vi "CRYCheck Statistic Data.vi"(8 "Results":string[](array[string]), 9 "Curves":string[](array[string]), 11 "No.VI":i32) -> (0 "Result Out":T1[](array[typedef]) {"Margin" format="%.2f"}, 2 "Data Out":T2 {"Z data" items=["dB", "Lin"]; "X data" items=["dB", "Lin"]; "Y data" items=["dB", "Lin"]; "Z dB ref" format="%.1f"; "Z axis" items=["Log", "Lin"]; "X dB ref" format="%.1f"; "X axis" items=["Log", "Lin"]; "Y axis" items=["Log", "Lin"]; "Y dB ref" format="%.1f"; "Curve"."z" format="%.2f"; "Curve"."y" format="%.2f"; "Curve"."x" format="%.2f"})   [LabVIEW 2013]
uses:
  Typedef Control/CRYData Cluster Array.ctl
  Typedef Control/CRYData Cluster.ctl
  Typedef Control/CRYResult Cluster.ctl
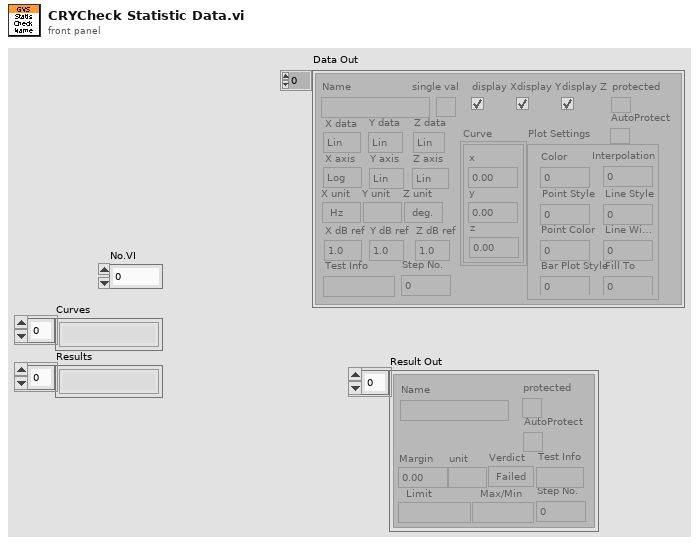
[diagram p1: front panel]
types:
  T1 = typedef "CRYResult Cluster.ctl" = cluster{"Name":string, "Margin":dbl, "unit":string, "Verdict":bool, "Limit":string, "Max/Min":string, "protected":bool, "Step No.":i32, "Test Info":string, "AutoProtect":bool}
  T2 = typedef "CRYData Cluster Array.ctl" = T3[]
  T3 = typedef "CRYData Cluster.ctl" = cluster{"Name":string, "Curve":cluster{"x":dbl, "y":dbl, "z":dbl}[], "X data":u16, "Y data":u16, "Z data":u16, "X axis":u16, "Y axis":u16, "Z axis":u16, "X unit":string, "Y unit":string, "Z unit":string, "X dB ref":dbl, "Y dB ref":dbl, "Z dB ref":dbl, "single val":bool, "protected":bool, "display X":bool, "display Y":bool, "display Z":bool, "Test Info":string, "Step No.":i32, "Plot Settings":cluster{"Color":u32, "Interpolation":u8, "Point Style":u8, "Line Style":u8, "Point Color":u32, "Line Width":u8, "Bar Plot Style":u8, "Fill To":i16}, "AutoProtect":bool}
  T4 = typedef "CRYResult Cluster Array.ctl" = T1[]
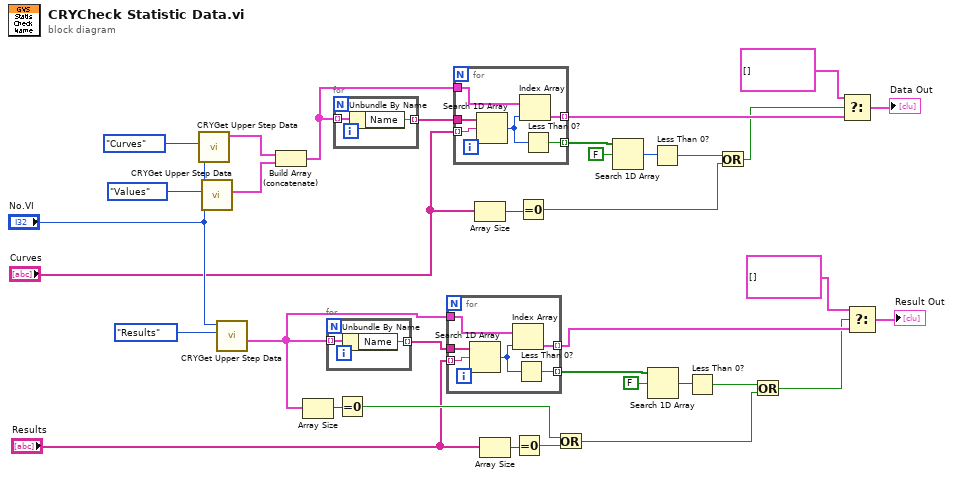
[diagram p0: block diagram]
diagram:
  n1 = call "CRYGet Upper Step Data.vi"("Type In"=enum16{"Curves", "Values", "Results", "WFM"}."Curves", "No.VI"="No.VI") -> ("Curve array"=w29:T2)  [unwired: 9 out]
  n2 = call "CRYGet Upper Step Data.vi"("Type In"=enum16{"Curves", "Values", "Results", "WFM"}."Values", "No.VI"="No.VI") -> ("Value array"=w28:T2)  [unwired: 9 out]
  n3 = call "CRYGet Upper Step Data.vi"("Type In"=enum16{"Curves", "Values", "Results", "WFM"}."Results", "No.VI"="No.VI") -> ("Result array"=w11:T4)  [unwired: 9 out]
  n4 = Build Array (concatenate)(w29, w28) -> (w26:T2)
  n5 = Array Size(array=w11) -> (size(s)=w12:i32)
  n6 = for {
    tunnel: w11 -> [w37] mode=indexing
    tunnel: [w36] -> w10 mode=indexing
    n7 = Unbundle By Name(w37) -> ("Name"=w36:string)
  }
  n8 = for {
    tunnel: w26 -> [w39] mode=indexing
    tunnel: [w38] -> w27 mode=indexing
    n9 = Unbundle By Name(w39) -> ("Name"=w38:string)
  }
  n10 = Equal To 0?(x=w12) -> (x = 0?=w13:bool)
  n11 = for {
    tunnel: "Results" -> [w45] mode=indexing
    tunnel: w10 -> [w44]
    tunnel: w11 -> [w43]
    tunnel: [w42] -> w4 mode=indexing
    tunnel: [w40] -> w5 mode=indexing
    n12 = Search 1D Array(1D array=w44, element=w45) -> (index of element=w41:i32)  [unwired: 1 in]
    n13 = Index Array(array=w43, index=w41) -> (element=w42:T1)
    n14 = Less Than 0?(x=w41) -> (x < 0?=w40:bool)
  }
  n15 = for {
    tunnel: "Curves" -> [w51] mode=indexing
    tunnel: w27 -> [w50]
    tunnel: w26 -> [w49]
    tunnel: [w48] -> w34 mode=indexing
    tunnel: [w46] -> w22 mode=indexing
    n16 = Search 1D Array(1D array=w50, element=w51) -> (index of element=w47:i32)  [unwired: 1 in]
    n17 = Index Array(array=w49, index=w47) -> (element=w48:T3)
    n18 = Less Than 0?(x=w47) -> (x < 0?=w46:bool)
  }
  n19 = Array Size(array="Curves") -> (size(s)=w16:i32)
  n20 = Array Size(array="Results") -> (size(s)=w15:i32)
  n21 = Equal To 0?(x=w15) -> (x = 0?=w14:bool)
  n22 = Equal To 0?(x=w16) -> (x = 0?=w7:bool)
  n23 = Or(x=w13, y=w14) -> (x .or. y?=w6:bool)
  n24 = Search 1D Array(1D array=w22, element=FALSE) -> (index of element=w24:i32)  [unwired: 1 in]
  n25 = Search 1D Array(1D array=w5, element=FALSE) -> (index of element=w20:i32)  [unwired: 1 in]
  n26 = Less Than 0?(x=w24) -> (x < 0?=w23:bool)
  n27 = Less Than 0?(x=w20) -> (x < 0?=w21:bool)
  n28 = Or(x=w23, y=w7) -> (x .or. y?=w18:bool)
  n29 = Or(x=w21, y=w6) -> (x .or. y?=w3:bool)
  n30 = Select(t=T2 [] ("Data in"), s=w18, f=w34) -> (s? t:f=→"Data Out":T2)
  n31 = Select(t=T1[] [], s=w3, f=w4) -> (s? t:f=→"Result Out":T1[])
